vi "gds_demod.vi"(8 "error in (no error)":errorcluster, 10 "input complex waveform":T3={"t0"=0.0, "dt"=1.0, "Y"=[]} caption="Received Signal" {"Y" format="%.3f"; "dt" format="%^.2e"; "t0" format="%.4f"}, 11 "Modulation Parameters":T1) -> (0 "error out":errorcluster, 1 "Measurements":T2 caption="measurements" {"FSK error (Hz)" format="%.2f"; "deviation error (Hz)" format="%.2f"; "frequency drift (Hz)" format="%.2f"; "frequency offset (Hz)" format="%.2f"}, 2 "output bit stream":i8[](array[numeric]) caption="Recovered Bits", 3 "Modulation Parameters Out":T1, 4 "recovered complex waveform":T3 {"Y" format="%.3f"; "dt" format="%^.2e"; "t0" format="%.4f"})   [LabVIEW 2012]
uses:
  <vilib>/addons/Modulation/Analog/controls/Complex Data Waveform.ctl
  <vilib>/addons/Modulation/Digital/General/MT Generate FSK System Parameters(M).vi
  <vilib>/addons/Modulation/Digital/General/MT Generate FSK Synchronization Parameters (bit array).vi
  <vilib>/addons/Modulation/Digital/General/MT Generate ASK system parameters (M).vi
  <vilib>/addons/Modulation/Digital/General/MT Generate ASK Synchronization Parameters (bit array).vi
  <vilib>/addons/Modulation/niDMT.lvlib
  <vilib>/addons/Modulation/niAMT.lvlib
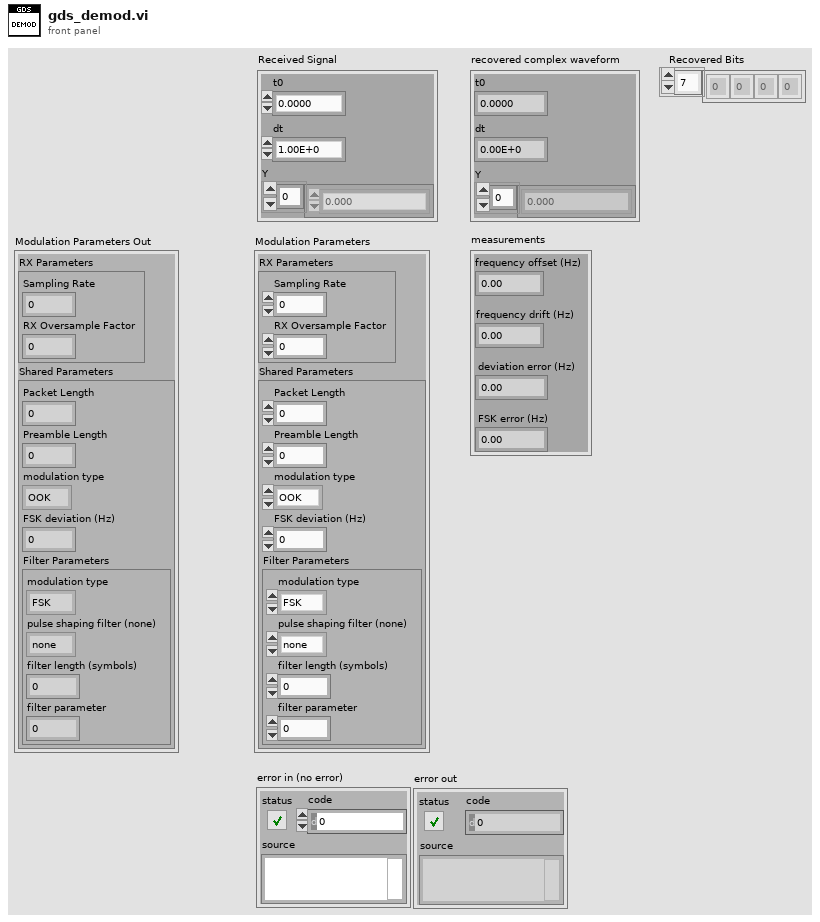
[diagram p1: front panel]
types:
  T1 = cluster{"RX Parameters":cluster{"Sampling Rate":dbl, "RX Oversample Factor":i32}, "Shared Parameters":cluster{"Packet Length":i32, "Preamble Length":i32, "modulation type":enum16{"OOK", "FSK", "PSK", "QAM", "MSK", "PAM", "ASK", "CPM"}, "FSK deviation (Hz)":dbl, "Filter Parameters":cluster{"modulation type":enum16{"FSK", "PSK", "QAM", "MSK", "PAM", "ASK", "CPM"}, "pulse shaping filter (none)":enum16{"none", "Raised Cosine", "Root Raised Cos", "Gaussian"}, "filter length (symbols)":i32, "filter parameter":dbl}}}
  T2 = cluster{"frequency offset (Hz)":dbl, "frequency drift (Hz)":dbl, "deviation error (Hz)":dbl, "FSK error (Hz)":dbl}
  T3 = typedef "niAMT.lvlib/Complex Data Waveform.ctl" = cluster{"t0":dbl, "dt":dbl, "Y":cdb[]}
  T4 = enum16{"OOK", "FSK", "PSK", "QAM", "MSK", "PAM", "ASK", "CPM"}
  T5 = enum16{"FSK", "PSK", "QAM", "MSK", "PAM", "ASK", "CPM"}
  T6 = enum16{"none", "Raised Cosine", "Root Raised Cos", "Gaussian"}
  T7 = cluster{"samples per symbol (16)":i32, "symbol map":dbl[], "symbol phase continuity":enum16{"continuous", "discontinuous"}}
  T8 = cluster{"expected sync location (symbols)":i32, "sync sequence":cdb[], "sync location uncertainty (symbols)":i32, "sync indent (symbols)":i32}
  T9 = cluster{"samples per symbol (16)":i32, "symbol map":cdb[]}
  T10 = cluster{"frequency offset (Hz)":dbl, "frequency drift (Hz)":dbl, "phase offset (deg)":dbl}
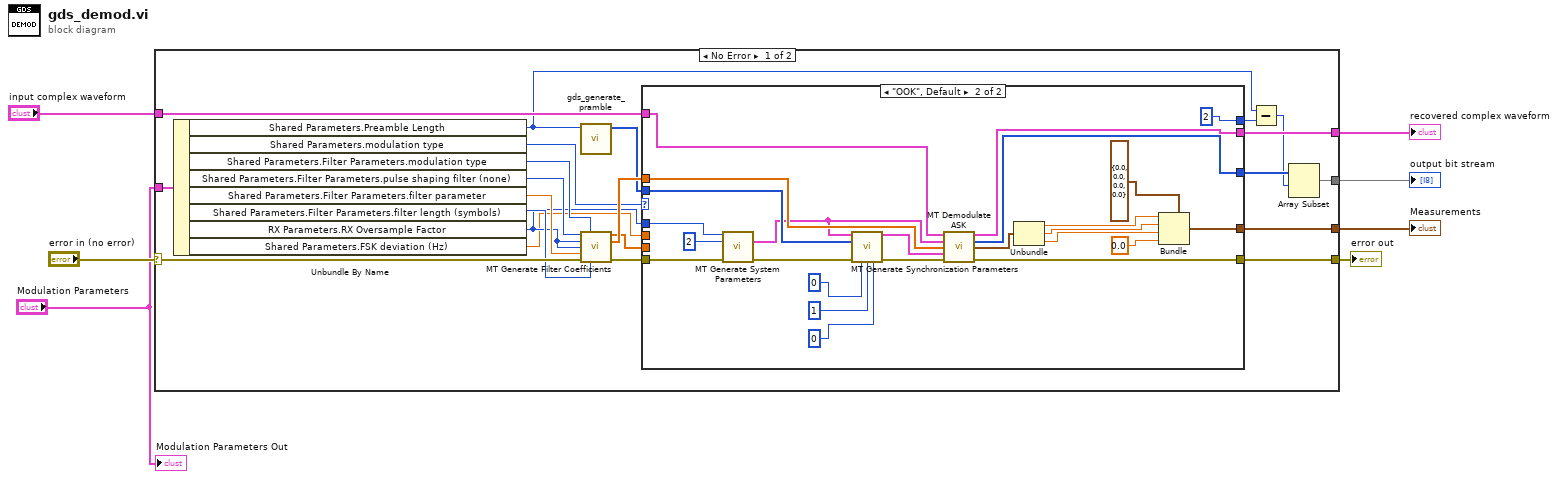
[diagram p0: block diagram]
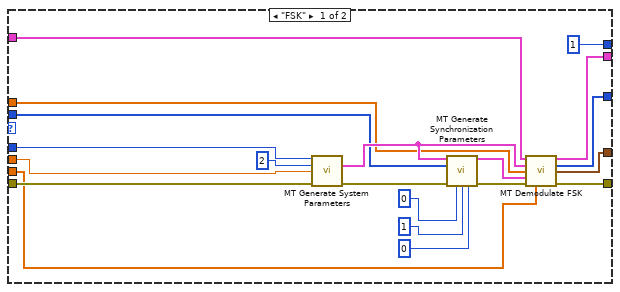
[diagram p2: hidden frame]
diagram:
  n1 = case shown="No Error" "error in (no error)" {
    selector: "error in (no error)" -> [w21 w75]
    tunnel: [w28 w75] -> w6
    tunnel: "input complex waveform" -> [w29 w74]
    tunnel: [w26 w74] -> w4
    tunnel: [w24 _] -> w3
    tunnel: [w17 _] -> w2
    tunnel: "Modulation Parameters" -> [w16 _]
    frame No Error {
      n2 = Unbundle By Name(w16) -> ("Shared Parameters.Preamble Length"=w9:i32, "Shared Parameters.modulation type"=w15:T4, "Shared Parameters.Filter Parameters.modulation type"=w14:T5, "Shared Parameters.Filter Parameters.pulse shaping filter (none)"=w13:T6, "Shared Parameters.Filter Parameters.filter parameter"=w12:dbl, "Shared Parameters.Filter Parameters.filter length (symbols)"=w11:i32, "RX Parameters.RX Oversample Factor"=w10:i32, "Shared Parameters.FSK deviation (Hz)"=w8:dbl)
      n3 = call "gds_generate_pramble.vi"("Preamble Length (bits)"=w9) -> ("Preamble"=w22:i32[])  [unwired: 10 in]
      n4 = call <vilib>:"MT Generate Filter Coefficients.vi"("pulse shaping filter (none)"=w13, "modulation type"=w14, "pulse shaping samples per symbol (16)"=w10, "matched samples per symbol (16)"=w10, "filter parameter"=w12, "error in (no error)"=w21, "filter length (symbols)"=w11) -> ("pulse shaping filter coefficients"=w19:dbl[], "matched filter coefficients"=w27:dbl[], "error out"=w20:errorcluster)  [unwired: 6 in]
      n5 = case shown="\"OOK\", Default" w15 {
        tunnel: w29 -> [w41 w73]
        tunnel: [w33 w72] -> w28
        tunnel: w10 -> [w38 w71]
        tunnel: w27 -> [w39 w70]
        tunnel: [w35 w69] -> w26
        tunnel: [w34 w68] -> w25
        tunnel: w22 -> [w40 w67]
        tunnel: w20 -> [w37 w60]
        tunnel: w19 -> [w36 _]
        tunnel: [1 ("y") 2 ("y")] -> w18
        tunnel: [w31 w51] -> w17
        tunnel: w8 -> [w30 _]
        frame "FSK" {
          n6 = call-poly <vilib>:"MT Generate System Parameters.vi"("samples per symbol (16)"=w38, "M-FSK (2)"=2 ("M-ASK (2)"), "FSK deviation (Hz)"=w30, "error in (no error)"=w37) -> ("FSK system parameters"=w49:T7, "error out"=w48:errorcluster)  [unwired: 9 in, 1 out]
          n7 = call-poly <vilib>:"MT Generate Synchronization Parameters.vi"("FSK system parameters"=w49, "sync bits"=w40, "error in (no error)"=w48, "expected sync location (symbols)"=0, "sync location uncertainty (symbols)"=1, "sync indent (symbols)"=0) -> ("FSK synchronization parameters"=w47:T8, "error out"=w43:errorcluster)  [unwired: 8 in]
          n8 = call <vilib>:"MT Demodulate FSK.vi"("input complex waveform"=w41, "FSK system parameters"=w49, "matched filter coefficients"=w39, "synchronization parameters"=w47, "error in (no error)"=w43, "pulse shaping filter coefficients"=w36) -> ("recovered complex waveform"=w35:T3, "output bit stream"=w34:i8[], "measurements"=w31:T2, "error out"=w33:errorcluster)  [unwired: 5 in, 1 out]
        }
        frame "OOK", Default {
          n9 = call-poly <vilib>:"MT Generate System Parameters.vi"("samples per symbol (16)"=w71, "M-ASK (2)"=2, "error in (no error)"=w60) -> ("ASK system parameters"=w66:T9, "error out"=w65:errorcluster)  [unwired: 10 in, 1 out]
          n10 = call-poly <vilib>:"MT Generate Synchronization Parameters.vi"("ASK system parameters"=w66, "sync bits"=w67, "error in (no error)"=w65, "expected sync location (symbols)"=0, "sync location uncertainty (symbols)"=1, "sync indent (symbols)"=0) -> ("ASK synchronization parameters"=w64:T8, "error out"=w59:errorcluster)  [unwired: 8 in]
          n11 = call <vilib>:"MT Demodulate ASK.vi"("input complex waveform"=w73, "ASK system parameters"=w66, "matched filter coefficients"=w70, "synchronization parameters"=w64, "error in (no error)"=w59) -> ("recovered complex waveform"=w69:T3, "output bit stream"=w68:i8[], "measurements"=w56:T10, "error out"=w72:errorcluster)  [unwired: 6 in, 1 out]
          n12 = Unbundle(w56) -> ("frequency offset (Hz)"=w55:dbl, "frequency drift (Hz)"=w54:dbl, "phase offset (deg)"=w53:dbl)
          n13 = Bundle(cluster=T2 {"frequency offset (Hz)"=0.0, "frequency drift (Hz)"=0.0, "deviation error (Hz)"=0.0, "FSK error (Hz)"=0.0} ("measurements"), "frequency offset (Hz)"=w55, "frequency drift (Hz)"=w54, "deviation error (Hz)"=w53, "FSK error (Hz)"=0.0) -> (w51:T2)
        }
      }
      n14 = Subtract(x=w9, y=w18) -> (x-y=w23:i32)
      n15 = Array Subset(array=w25, index=w23) -> (w24:i8[])  [unwired: 1 in]
    }
    frame Error {
    }
  }
  "error out" <- w6
  "recovered complex waveform" <- w4
  "output bit stream" <- w3
  "Measurements" <- w2
  "Modulation Parameters Out" <- "Modulation Parameters"
